vi "_write.vi"(8 "Error in (no error)":errorcluster, 10 "Log in":T1 {"Priority" items=["EMERGENCY", "ALERT", "CRITICAL", "ERROR", "WARNING", "NOTICE", "INFO", "DEBUG"]}, 11 "LogWriterEmail in":refnum<class "LogWriterEmail.lvclass">) -> (0 "Error out":errorcluster, 3 "LogWriterEmail out":refnum<class "LogWriterEmail.lvclass">)   [LabVIEW 2011, in "LogWriterEmail.lvclass"]
uses:
  LogWriterEmail.lvclass
  Log/LogCluster.ctl
  Log/PrioritiesRing.ctl
  LogWriterEmail.lvclass/LogWriterEmail.ctl
  LogWriterMock/LogWriterMock.lvclass
  Log/Log.lvclass
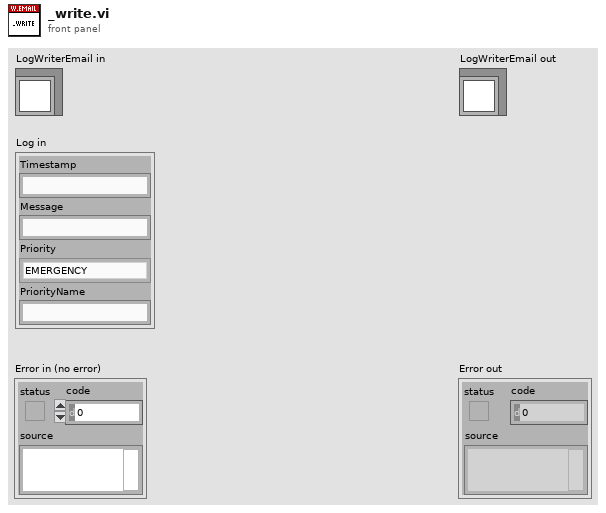
[diagram p1: front panel]
types:
  T1 = typedef "Log.lvclass/LogCluster.ctl" = cluster{"Timestamp":string, "Message":string, "Priority":T2, "PriorityName":string}
  T2 = typedef "Log.lvclass/PrioritiesRing.ctl" = u32
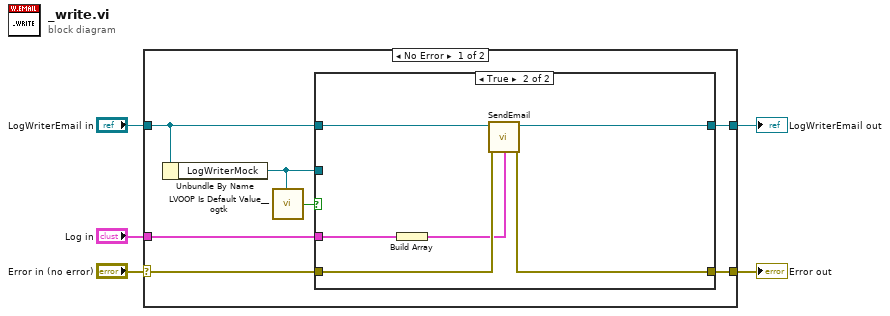
[diagram p0: block diagram]
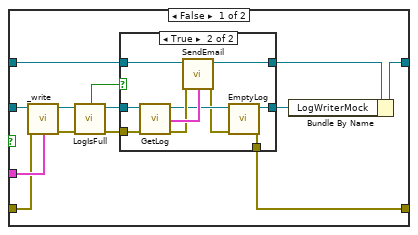
[diagram p2: hidden frame]
diagram:
  n1 = case shown="No Error" "Error in (no error)" {
    selector: "Error in (no error)" -> [w7 w46]
    tunnel: [w6 w46] -> w4
    tunnel: [w9 w45] -> w2
    tunnel: "LogWriterEmail in" -> [w10 w45]
    tunnel: "Log in" -> [w11 _]
    frame No Error {
      n2 = Unbundle By Name(w10) -> ("LogWriterMock"=w8:refnum<class "LogWriterMock.lvclass">)
      n3 = call <userlib>:"LVOOP Is Default Value__ogtk.vi"("Object"=w8) -> ("Is Default Value?"=w12:bool)
      n4 = case shown="True" w12 {
        tunnel: w11 -> [w24 w40]
        tunnel: w10 -> [w17 w44]
        tunnel: [w13 w43] -> w9
        tunnel: w8 -> [w25 _]
        tunnel: w7 -> [w23 w42]
        tunnel: [w16 w41] -> w6
        frame False {
          n5 = call-dynamic "_write.vi"("Error in (no error)"=w23, "Log in"=w24, "LogWriterMock in"=w25) -> ("Error out"=w21:errorcluster, "LogWriterMock out"=w22:refnum<class "LogWriterMock.lvclass">)  [unwired: 7 in]
          n6 = call "LogIsFull.vi"("Error in (no error)"=w21, "LogWriterMock in"=w22) -> ("Error out"=w18:errorcluster, "BufferIsFull"=w20:bool, "LogWriterMock out"=w19:refnum<class "LogWriterMock.lvclass">)  [unwired: 7 in]
          n7 = case shown="True" w20 {
            tunnel: w19 -> [w26 w38]
            tunnel: w18 -> [w27 w37]
            tunnel: w17 -> [w28 w36]
            tunnel: [w28 w35] -> w14
            tunnel: [w26 w30] -> w15
            tunnel: [w27 w29] -> w16
            frame False {
            }
            frame True {
              n8 = call "GetLog.vi"("Error in (no error)"=w37, "LogWriterMock in"=w38) -> ("Error out"=w33:errorcluster, "Array log out"=w34:T1[], "LogWriterMock out"=w32:refnum<class "LogWriterMock.lvclass">)  [unwired: 7 in]
              n9 = call "SendEmail.vi"("Error in (no error)"=w33, "Array log in"=w34, "LogWriterEmail in"=w36) -> ("Error out"=w31:errorcluster, "LogWriterEmail out"=w35:refnum<class "LogWriterEmail.lvclass">)  [unwired: 7 in]
              n10 = call "EmptyLog.vi"("Error in (no error)"=w31, "LogWriterMock in"=w32) -> ("Error out"=w29:errorcluster, "LogWriterMock out"=w30:refnum<class "LogWriterMock.lvclass">)  [unwired: 8 in]
            }
          }
          n11 = Bundle By Name(cluster=w14, "LogWriterMock"=w15) -> (w13:refnum<class "LogWriterEmail.lvclass">)
        }
        frame True {
          n12 = Build Array(w40) -> (w39:T1[])
          n13 = call "SendEmail.vi"("Error in (no error)"=w42, "Array log in"=w39, "LogWriterEmail in"=w44) -> ("Error out"=w41:errorcluster, "LogWriterEmail out"=w43:refnum<class "LogWriterEmail.lvclass">)  [unwired: 7 in]
        }
      }
    }
    frame Error {
    }
  }
  "Error out" <- w4
  "LogWriterEmail out" <- w2
